vi "SEQ Add sequence step.vi"(8 "error in (no error)":errorcluster, 10 "seq.new step":T2, 11 "Refnum in":refnum<k20>) -> (0 "error out":errorcluster, 3 "Refnum out":T1)   [LabVIEW 2019, in "FPGA sequencer API.lvlib"]
uses:
  FPGA sequencer API.lvlib
  FPGA sequencer ref.ctl
  <vilib>/Utility/error.llb/Error Cluster From Error Code.vi
  <vilib>/rvi/errors/niLvFpgaAdjustHostInterfaceError.vi
  <vilib>/rvi/interface/nirviReadWriteControl/nirviReadWriteControl.xnode
  NiFpgaLv.dll
  <vilib>/rvi/interface/Simulation/niFpgaSimulationCallBeginRW.vi
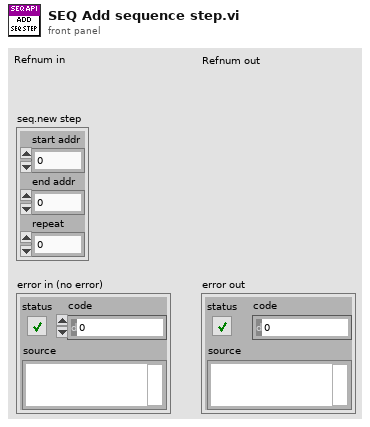
[diagram p1: front panel]
types:
  T1 = typedef "FPGA sequencer API.lvlib/FPGA sequencer ref.ctl" = refnum<k20>
  T2 = cluster{"start addr":u32, "end addr":u32, "repeat":u64}
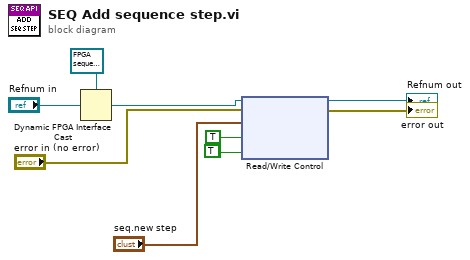
[diagram p0: block diagram]
diagram:
  (unwired) TRUE ("seq.rst")
  n1 = Dynamic FPGA Interface Cast(Session In=T1 refnum ("FPGA VI Reference Out"), Type="Refnum in") -> (Session Out=w2:T1)
  n2 = xnode "Read/Write Control"("FPGA VI Reference In"=w2, "error in"="error in (no error)", "seq.new step"="seq.new step", "seq.add step"=TRUE ("seq.rst"), "seq.add step"=FALSE ("seq.rst")) -> ("FPGA VI Reference Out"=→"Refnum out":T1, "error out"=→"error out":errorcluster)
